vi "GVmotor_read_Pot_V0.vi"(8 "file_name":string="Pot_V0.txt") -> (3 "V0":dbl)   [LabVIEW 2019]
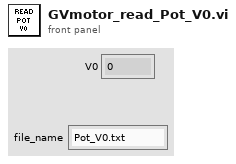
[diagram p1: front panel]
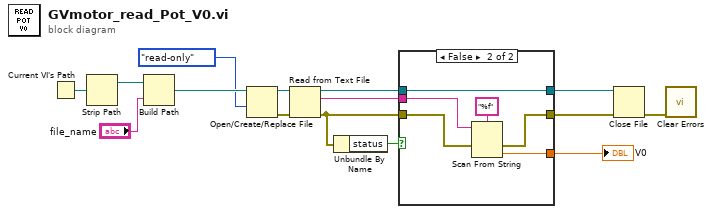
[diagram p0: block diagram]
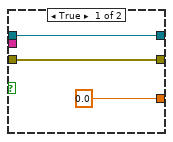
[diagram p2: hidden frame]
diagram:
  n1 = Current VI's Path() -> (path=w13:path)
  n2 = Strip Path(path=w13) -> (stripped path=w12:path)  [unwired: 1 out]
  n3 = Build Path(base path=w12, name or relative path="file_name") -> (appended path=w11:path)
  n4 = Open/Create/Replace File(file path (use dialog)=w11, access (0:read/write)=enum16{"read/write", "read-only", "write-only"}."read-only") -> (refnum out=w14:refnum<file>, error out=w8:errorcluster)  [unwired: 4 in, 1 out]
  n5 = Read from Text File(file (use dialog)=w14, error in=w8) -> (refnum out=w4:refnum<file>, text=w15:string, error out=w5:errorcluster)  [unwired: 2 in, 1 out]
  n6 = Unbundle By Name(w5) -> ("status"=w2:bool)
  n7 = case shown="False" w2 {
    tunnel: w15 -> [_ w24]
    tunnel: [w17 w22] -> w7
    tunnel: [0.0 w21] -> w6
    tunnel: w5 -> [w17 w20]
    tunnel: w4 -> [w18 w19]
    tunnel: [w18 w19] -> w3
    frame True {
    }
    frame False {
      n8 = Scan From String(format string="%f", input string=w24, error in=w20) -> (error out=w22:errorcluster, output 1=w21:dbl)  [unwired: 2 in, 2 out]
    }
  }
  "V0" <- w6
  n9 = Close File(refnum=w3, error in=w7) -> (error out=w1:errorcluster)  [unwired: 1 out]
  n10 = call <vilib>:"Clear Errors.vi"("error in (no error)"=w1) -> ()  [unwired: 5 in, 2 out]
